vi "UpdateLotTable_New.vi"(8 "error in (no error)":errorcluster, 10 "input cluster":T1 {"50mA Data"."Reverse" format="%#_3g"; "50mA Data"."Current,mA" format="%_6g"; "50mA Data"."Knee Current" format="%#_3g"; "50mA Data"."WL" format="%_6g"; "50mA Data"."Voltage" format="%_6g"; "50mA Data"."Power" format="%_5g"; "20mA Data"."Reverse" format="%#_3g"; "20mA Data"."Current,mA" format="%_6g"; "20mA Data"."Knee Current" format="%#_3g"; "20mA Data"."WL" format="%_6g"; "20mA Data"."Voltage" format="%_6g"; "20mA Data"."Power" format="%_5g"}, 11 "LotData in":refnum<class "LotData.lvclass">) -> (0 "error out":errorcluster, 3 "LotData out":refnum<class "LotData.lvclass">)   [LabVIEW 2012, in "LotData.lvclass"]
uses:
  LotData.lvclass
  Controls/TestData.ctl
  Controls/Measurement.ctl
  LotData.lvclass/LotData.ctl
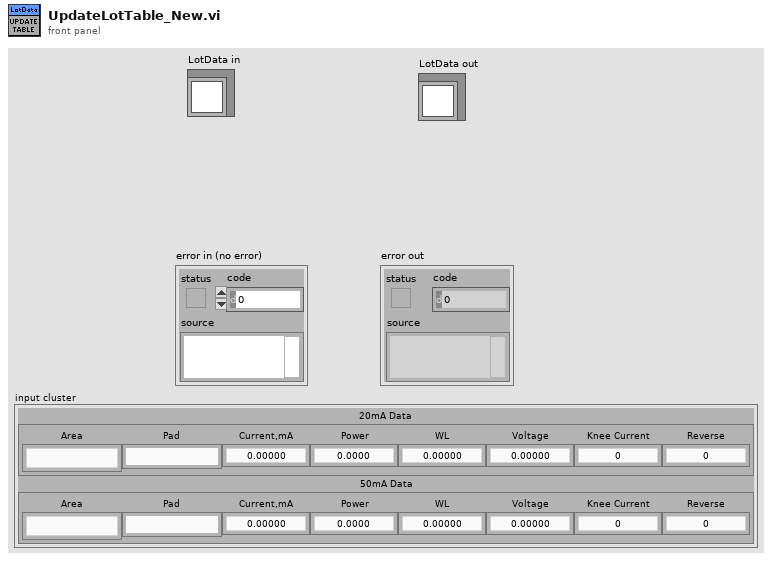
[diagram p1: front panel]
types:
  T1 = typedef "TestData.ctl" = cluster{"20mA Data":T2, "50mA Data ":T2}
  T2 = typedef "Measurement.ctl" = cluster{"Area":string, "Pad":string, "Current,mA":dbl, "Power":dbl, "WL":dbl, "Voltage":dbl, "Knee Current":dbl, "Reverse":dbl}
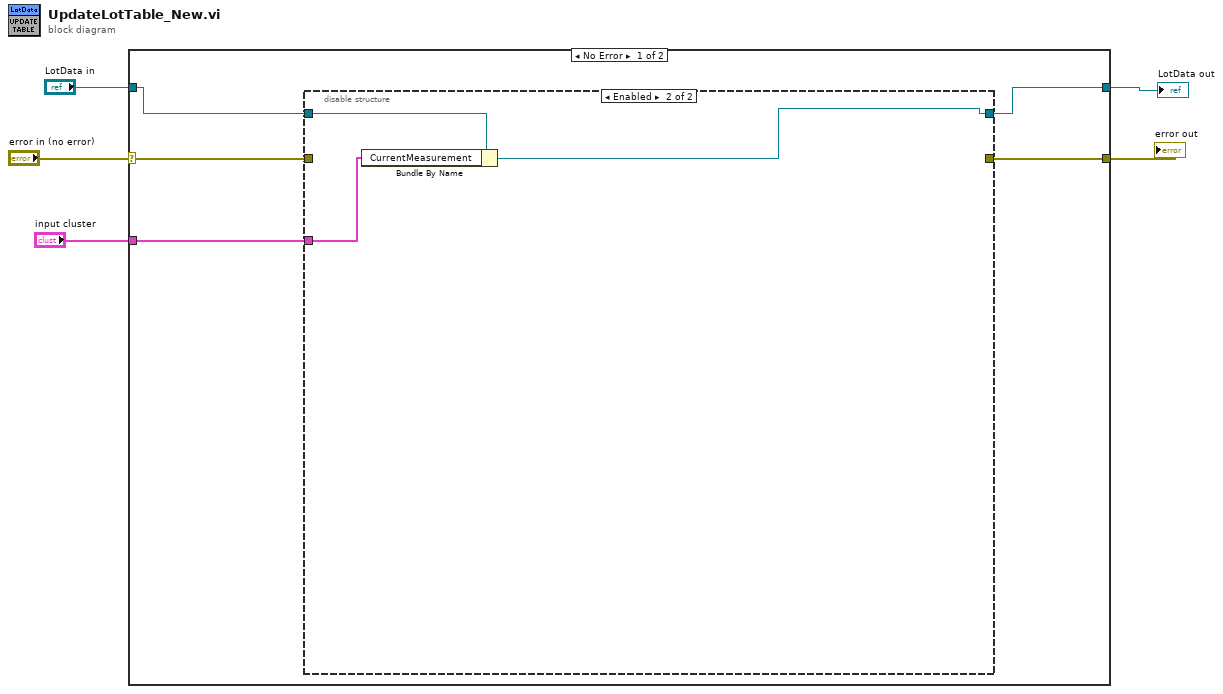
[diagram p0: block diagram]
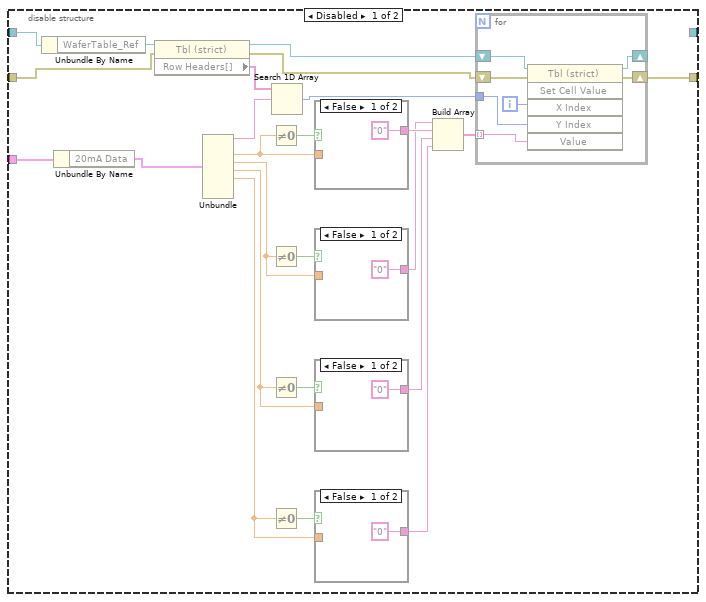
[diagram p2: hidden frame]
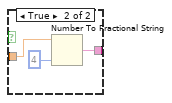
[diagram p3: hidden frame]
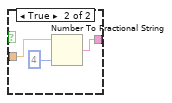
[diagram p4: hidden frame]
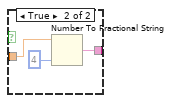
[diagram p5: hidden frame]
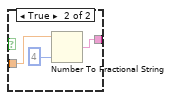
[diagram p6: hidden frame]
diagram:
  n1 = case shown="No Error" "error in (no error)" {
    selector: "error in (no error)" -> [w7 w62]
    tunnel: [w10 w62] -> w4
    tunnel: [w6 w61] -> w2
    tunnel: "LotData in" -> [w9 w61]
    tunnel: "input cluster" -> [w8 _]
    frame No Error {
      n2 = disable-structure shown="Enabled" {
        disable-tunnel: [w33 _] -> w10
        disable-tunnel: w9 -> [w32 w60]
        disable-tunnel: w8 -> [w13 w59]
        disable-tunnel: w7 -> [w12 _]
        disable-tunnel: [_ w58] -> w6
        frame Disabled {
          n3 = Unbundle By Name(w32) -> ("WaferTable_Ref"=w34:refnum<vi>)
          n4 = Unbundle By Name(w13) -> ("20mA Data"=w31:T2)
          n5 = property class="Tbl (strict)"(reference=w34, error in=w12) -> (reference out=w28:refnum<vi>, error out=w11:errorcluster, "Row Headers[]"=w30:string[])
          n6 = Unbundle(w31) -> ("Area"=w29:string, "Current,mA"=w24:dbl, "Power"=w18:dbl, "WL"=w19:dbl, "Voltage"=w20:dbl)  [unwired: 3 out]
          n7 = Not Equal To 0?(x=w24) -> (x != 0?=w25:bool)
          n8 = Not Equal To 0?(x=w18) -> (x != 0?=w23:bool)
          n9 = Not Equal To 0?(x=w19) -> (x != 0?=w22:bool)
          n10 = Not Equal To 0?(x=w20) -> (x != 0?=w21:bool)
          n11 = Search 1D Array(1D array=w30, element=w29) -> (index of element=w27:i32)  [unwired: 1 in]
          n12 = case shown="False" w25 {
            tunnel: w24 -> [_ w50]
            tunnel: ["0" ("F-format string") w48] -> w17
            frame False {
            }
            frame True {
              n13 = Number To Fractional String(number=w50, precision (6)=i16 4) -> (F-format string=w48:string)  [unwired: 2 in]
            }
          }
          n14 = case shown="False" w23 {
            tunnel: ["0" ("F-format string") w45] -> w16
            tunnel: w18 -> [_ w44]
            frame False {
            }
            frame True {
              n15 = Number To Fractional String(number=w44, precision (6)=i16 4) -> (F-format string=w45:string)  [unwired: 2 in]
            }
          }
          n16 = case shown="False" w22 {
            tunnel: ["0" ("F-format string") w41] -> w15
            tunnel: w19 -> [_ w40]
            frame False {
            }
            frame True {
              n17 = Number To Fractional String(number=w40, precision (6)=i16 4) -> (F-format string=w41:string)  [unwired: 2 in]
            }
          }
          n18 = case shown="False" w21 {
            tunnel: ["0" ("F-format string") w37] -> w14
            tunnel: w20 -> [_ w36]
            frame False {
            }
            frame True {
              n19 = Number To Fractional String(number=w36, precision (6)=i16 4) -> (F-format string=w37:string)  [unwired: 2 in]
            }
          }
          n20 = Build Array(w16, w17, w15, w14) -> (w26:string[])
          n21 = for {
            tunnel: w26 -> [w54] mode=indexing
            tunnel: w27 -> [w56]
            shift-right: [w52] -> w33
            shift-left: w11 -> [w53]
            shift-right: [w51] -> _
            shift-left: w28 -> [w57]
            i -> [w55]
            n22 = invoke class="Tbl (strict)" method="Set Cell Value"(reference=w57, error in=w53, "X Index"=w55, "Y Index"=w56, "Value"=w54) -> (reference out=w51:refnum<vi>, error out=w52:errorcluster)  [unwired: 1 in, 4 out]
          }
        }
        frame Enabled {
          n23 = Bundle By Name(cluster=w60, "CurrentMeasurement"=w59) -> (w58:refnum<class "LotData.lvclass">)
        }
      }
    }
    frame Error {
    }
  }
  "error out" <- w4
  "LotData out" <- w2
